vi "add alarm.vi"(8 "error in":errorcluster, 10 "alarm name":string, 11 "alarms module configuration in":refnum<class "alarms module configuration.lvclass">) -> (0 "error out":errorcluster, 2 "created channels":refnum<class "TBM channel.lvclass">[](array[class]), 3 "alarms module configuration out":refnum<class "alarms module configuration.lvclass">)   [LabVIEW 2013, in "alarms module configuration.lvclass"]
uses:
  alarms module configuration.lvclass
  <vilib>/NI/Tag Bus Module Framework/channel/TBM channel.lvclass
  alarms module configuration.lvclass/alarms module configuration.ctl
  alarm configuration.ctl
  alarm comparison.ctl
  compare type.ctl
  boolean operation.ctl
  <vilib>/NI/Tag Bus/tag/Data Type.ctl
  <vilib>/NI/Tag Bus Module Framework/channel/channel classification.ctl
  <vilib>/NI/Tag Bus/tag/tag descriptor.lvclass
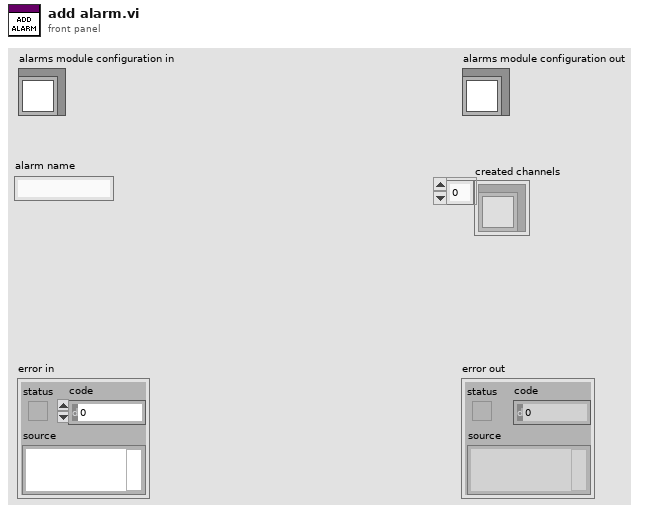
[diagram p1: front panel]
types:
  T1 = typedef "alarms module configuration.lvclass/alarm comparison.ctl" = cluster{"input channel":refnum<class "TBM channel.lvclass">, "limit":dbl, "comparison":T2}
  T2 = typedef "alarms module configuration.lvclass/compare type.ctl" = enum16{">", "<", ">=", "<=", "="}
  T3 = typedef "alarms module configuration.lvclass/boolean operation.ctl" = enum16{"AND", "OR"}
  T4 = typedef "TBM channel.lvclass/channel classification.ctl" = enum16{"input data", "output data", "processing parameter", "processing result"}
  T5 = typedef "alarms module configuration.lvclass/alarm configuration.ctl" = cluster{"alarm name":string, "comparisons":T1[], "unlatch":refnum<class "TBM channel.lvclass">, "output":refnum<class "TBM channel.lvclass">, "boolean op":T3}
  T6 = typedef "tag bus.lvlib/tag descriptor.lvclass/Data Type.ctl" = enum16{"Double", "Single", "I64", "I32", "I16", "I8", "U64", "U32", "U16", "U8", "Boolean", "String", "Array of Double", "Array of Single", "Array of I64", "Array of I32", "Array of I16", "Array of I8", "Array of U64", "Array of U32", "Array of U16", "Array of U8", "Array of Boolean", "Array of String"}
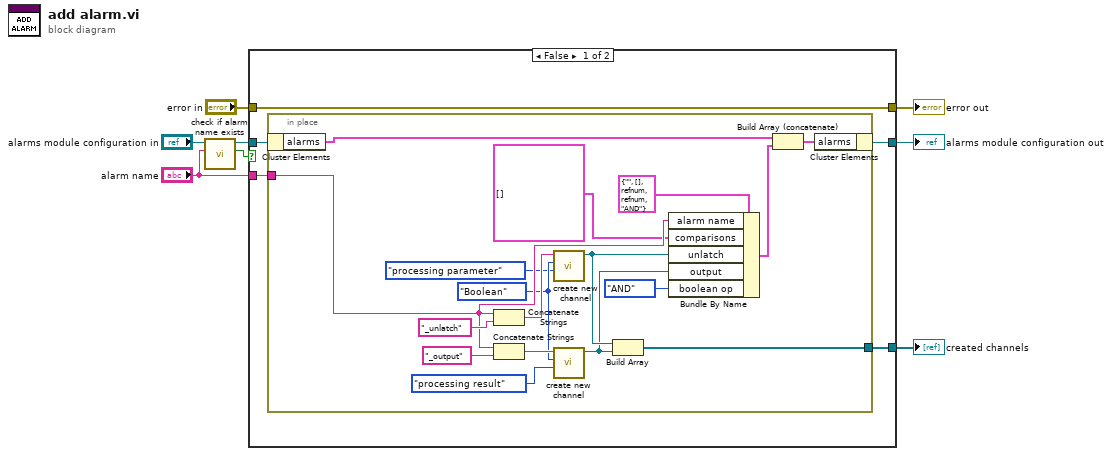
[diagram p0: block diagram]
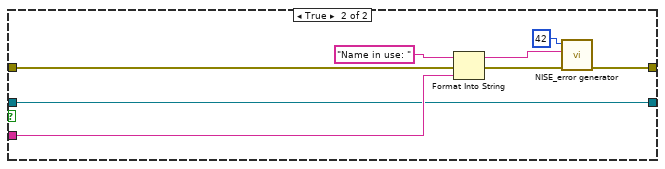
[diagram p2: hidden frame]
diagram:
  n1 = call "check if alarm name exists.vi"("name to locate"="alarm name", "alarms module configuration in"="alarms module configuration in") -> ("found?"=w5:bool, "alarms module configuration out"=w3:refnum<class "alarms module configuration.lvclass">)  [unwired: 7 in, 1 out]
  n2 = case shown="False" w5 {
    tunnel: [w11 w37] -> w7
    tunnel: "error in" -> [w11 w38]
    tunnel: "alarm name" -> [w10 w33]
    tunnel: [w12 w31] -> w4
    tunnel: w3 -> [w13 w31]
    tunnel: [w9 _] -> w2
    frame False {
      n3 = in-place {
        in-place-border: w10 -> [w22]
        in-place-border: [w14] -> w9
        w21 = Data_Type."Boolean" ("data type")
        n4 = in-place-cluster #1(w13) -> ("alarms"=w30:T5[])
        n5 = Concatenate Strings(w22, "_unlatch" ("string")) -> (w26:string)
        n6 = Concatenate Strings(w22, "_output" ("string")) -> (w23:string)
        n7 = call <vilib>:"create new channel.vi"("channel classification"=channel_classification."processing parameter", "data type"=w21, "channel name"=w26) -> ("channel"=w16:refnum<class "TBM channel.lvclass">)  [unwired: 8 in]
        n8 = call <vilib>:"create new channel.vi"("channel classification"=channel_classification."processing result", "data type"=w21, "channel name"=w23) -> ("channel"=w15:refnum<class "TBM channel.lvclass">)  [unwired: 8 in]
        n9 = Build Array(w16, w15) -> (w14:refnum<class "TBM channel.lvclass">[])
        n10 = Bundle By Name(cluster=T5 {"alarm name"="", "comparisons"=[], "unlatch"=refnum, "output"=refnum, "boolean op"=enum."AND"} ("alarm config"), "alarm name"=w22, "comparisons"=T1[] [], "unlatch"=w16, "output"=w15, "boolean op"=boolean_operation."AND") -> (w27:T5)
        n11 = Build Array (concatenate)(w30, w27) -> (w29:T5[])
        n12 = in-place-cluster #1("alarms"=w29) -> (w12:refnum<class "alarms module configuration.lvclass">)
      }
    }
    frame True {
      n13 = Format Into String(initial string="Name in use: " ("append error message"), error in=w38, w33) -> (resulting string=w32:string, error out=w35:errorcluster)  [unwired: 1 in]
      n14 = call <vilib>:"NISE_error generator.vi"("error in"=w35, "append error message"=w32, "error code (0)"=42) -> ("error out"=w37:errorcluster)  [unwired: 6 in]
    }
  }
  "error out" <- w7
  "alarms module configuration out" <- w4
  "created channels" <- w2
